vi "Invalidate Iteration.vi"(8 "error in (no error)":errorcluster, 11 "Transfer Group in":refnum<class "Transfer Group.lvclass">) -> (0 "error out":errorcluster, 3 "Transfer Group out":refnum<class "Transfer Group.lvclass">)   [LabVIEW 2017, in "DSF Core.lvlib" / "Transfer Group.lvclass"]
uses:
  Transfer Group.lvclass
  Transfer Group.lvclass/Transfer Group.ctl
  Timing/Timing.lvclass
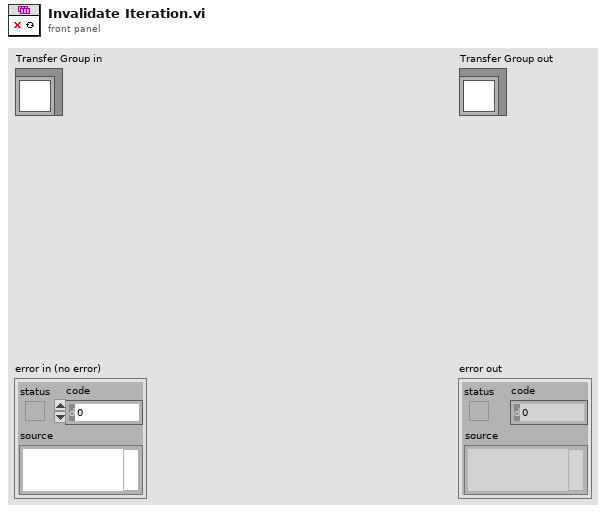
[diagram p1: front panel]
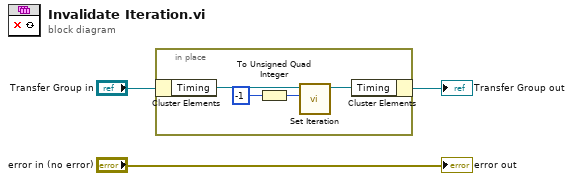
[diagram p0: block diagram]
diagram:
  n1 = in-place {
    n2 = in-place-cluster #1("Transfer Group in") -> ("Timing"=w7:refnum<class "Timing.lvclass">)
    n3 = To Unsigned Quad Integer(1:i64 -1 ("Iteration")) -> (0:w4:u64)
    n4 = call "Set Iteration.vi"("Iteration"=w4, "Timing in"=w7) -> ("Timing out"=w6:refnum<class "Timing.lvclass">)  [unwired: 9 in]
    n5 = in-place-cluster #1("Timing"=w6) -> (→"Transfer Group out":refnum<class "Transfer Group.lvclass">)
  }
  "error out" <- "error in (no error)"
